vi "FilterInfoFGV.vi"(1 "GetSet enum":T1, 2 "FilterInfo in":T2={"filter type"=enum."Lowpass", "high cutoff freq: fh"=0.45000000000000007, "low cutoff freq: fl"=0.12500000000000006, "order"=2} {"low cutoff freq: fl" format="%0.4f"; "high cutoff freq: fh" format="%0.2f"}) -> (0 "FilterInfo out":T2={"filter type"=enum."Lowpass", "high cutoff freq: fh"=0.45000000000000007, "low cutoff freq: fl"=0.12500000000000006, "order"=2} {"low cutoff freq: fl" format="%0.4f"; "high cutoff freq: fh" format="%0.2f"})   [LabVIEW 2016]
uses:
  Generation/Filter/FilterInfo.ctl
  <vilib>/Analysis/3filter.llb/Filter Passband Type.ctl
  FGV/GetSetEnum.ctl
  <vilib>/Analysis/NI_AALBase.lvlib
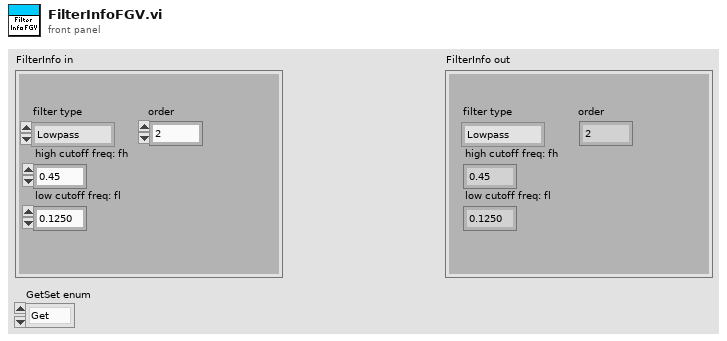
[diagram p1: front panel]
types:
  T1 = typedef "GetSetEnum.ctl" = enum16{"Get", "Set"}
  T2 = typedef "FilterInfo.ctl" = cluster{"filter type":T3, "high cutoff freq: fh":dbl, "low cutoff freq: fl":dbl, "order":i32}
  T3 = typedef "NI_AALBase.lvlib/Filter Passband Type.ctl" = enum32{"Lowpass", "Highpass", "Bandpass", "Bandstop"}
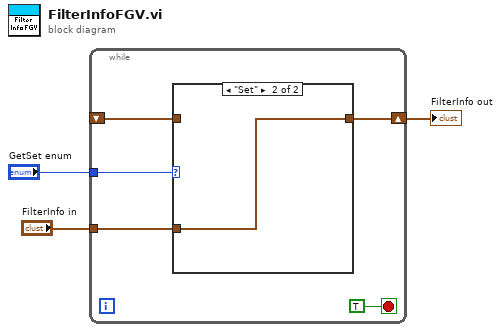
[diagram p0: block diagram]
diagram:
  n1 = while {
    tunnel: "GetSet enum" -> [w7]
    tunnel: "FilterInfo in" -> [w5]
    shift-right: [w6] -> w2
    shift-left: _ -> [w4]
    stop <- TRUE stop-if-true
    n2 = case shown="\"Set\"" w7 {
      tunnel: [w9 w10] -> w6
      tunnel: w5 -> [_ w10]
      tunnel: w4 -> [w9 _]
      frame "Get", Default {
      }
      frame "Set" {
      }
    }
  }
  "FilterInfo out" <- w2
